vi "Do Bar Sample Resistivity Calculations.vi"(8 "error in (no error)":errorcluster) -> (0 "error out":errorcluster)   [LabVIEW 2016, in "Hall Effect Library.lvlib"]
uses:
  Hall Effect Library.lvlib
  Global Variables/Hall Effect Data.vi
  Global Variables/Test Settings.vi
panel:
  out "p":dbl
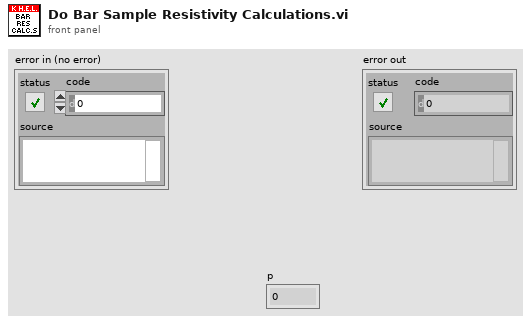
[diagram p1: front panel]
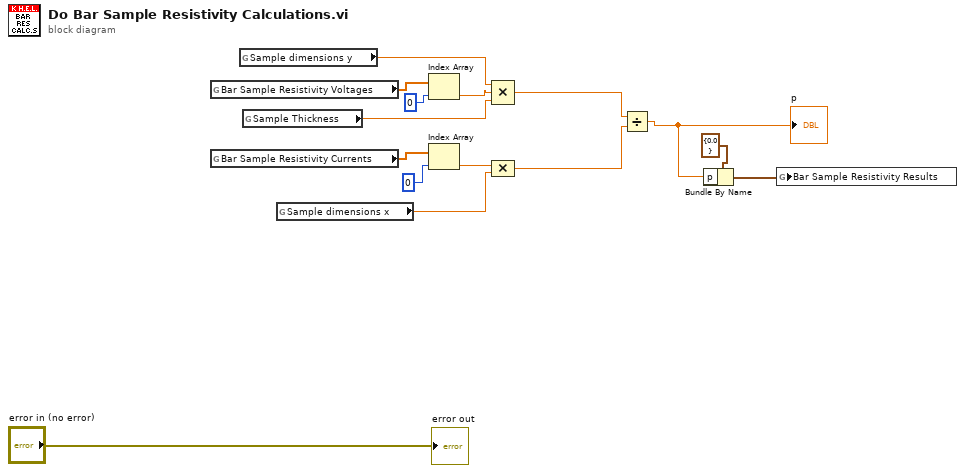
[diagram p0: block diagram]
diagram:
  n1 = global read "Hall Effect Data.vi" "Bar Sample Resistivity Voltages"() -> (w9:dbl[])
  n2 = global read "Hall Effect Data.vi" "Bar Sample Resistivity Currents"() -> (w6:dbl[])
  n3 = global read "Test Settings.vi" "Sample dimensions y"() -> (w14:dbl)
  n4 = global read "Test Settings.vi" "Sample Thickness"() -> (w13:dbl)
  n5 = global read "Test Settings.vi" "Sample dimensions x"() -> (w12:dbl)
  n6 = Index Array(array=w9, index=0) -> (element=w7:dbl)
  n7 = Index Array(array=w6, index=0) -> (element=w4:dbl)
  n8 = Compound Arithmetic op=MULTIPLY(w14, w7, w13) -> (w11:dbl)
  n9 = Compound Arithmetic op=MULTIPLY(w4, w12) -> (w10:dbl)
  n10 = Divide(x=w11, y=w10) -> (x/y=w3:dbl)
  "p" <- w3
  n11 = Bundle By Name(cluster=cluster{"p":dbl} {"p"=0.0} ("Bar Sample Resistivity Results"), "p"=w3) -> (w1:cluster{"p":dbl})
  n12 = global write "Hall Effect Data.vi" "Bar Sample Resistivity Results"(w1) -> ()
  "error out" <- "error in (no error)"
